vi "自动配置的串口通信组件(Master)vi.vi"(0 "查询":string(combo)="CH0", 5 "error in":errorcluster) -> (14 "读取缓冲区":string, 19 "error out":errorcluster)   [LabVIEW 2013]
uses:
  <vilib>/Instr/_visa.llb/VISA Configure Serial Port (Instr).vi
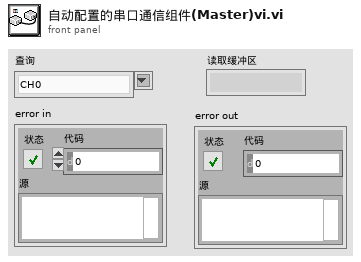
[diagram p1: front panel]
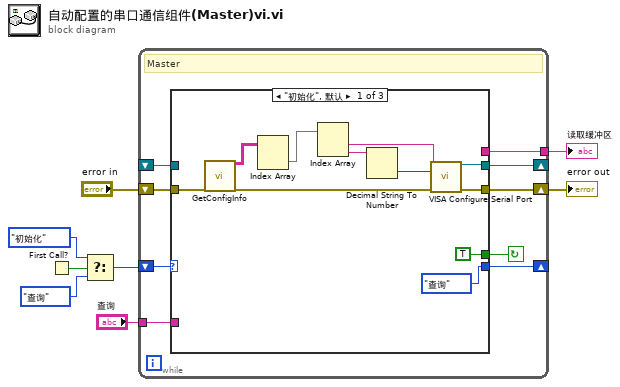
[diagram p0: block diagram]
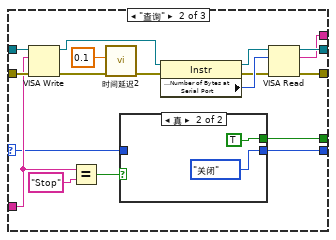
[diagram p2: hidden frame]
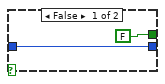
[diagram p3: hidden frame]
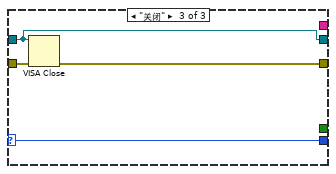
[diagram p4: hidden frame]
diagram:
  n1 = First Call?() -> (First Call?: T/F=w5:bool)
  n2 = Select(t=enum16{"初始化", "空闲", "查询", "关闭"}."初始化" ("枚举"), s=w5, f=enum16{"初始化", "空闲", "查询", "关闭"}."查询" ("枚举")) -> (s? t:f=w4:enum16{"初始化", "空闲", "查询", "关闭"})
  n3 = while {
    shift-right: [w17] -> w1
    shift-left: "error in" -> [w15]
    shift-right: [w16] -> _
    shift-left: _ -> [w14]
    tunnel: "查询" -> [w13]
    tunnel: [w12] -> w7
    shift-right: [w9] -> _
    shift-left: w4 -> [w10]
    stop <- w11 continue-if-true
    # "Master"
    n4 = case shown="\"初始化\", 默认" w10 {
      selector: w10 -> [_ w31 w51]
      tunnel: [w28 w37 w52] -> w16
      tunnel: [w27 w36 w53] -> w17
      tunnel: w15 -> [w24 w38 w54]
      tunnel: w14 -> [_ w39 w52]
      tunnel: w13 -> [_ w34 _]
      tunnel: [_ w35 _] -> w12
      tunnel: [TRUE w29 _] -> w11
      tunnel: [enum16{"初始化", "空闲", "查询", "关闭"}."查询" ("枚举") w30 w51] -> w9
      frame "初始化", Default {
        n5 = call "GetConfigInfo.vi"("error in (no error)"=w24) -> ("串口配置"=w23:string[][], "error out"=w18:errorcluster)  [unwired: 17 in]
        n6 = Index Array(array=w23) -> (element=w22:string[])  [unwired: 2 in]
        n7 = Index Array(array=w22) -> (element #1=w21:string, element #2=w20:string)  [unwired: 2 in]
        n8 = Decimal String To Number(string=w20) -> (number=w19:i32)  [unwired: 2 in, 1 out]
        n9 = call-poly "VISA Configure Serial Port"("VISA resource name"=w21, "baud rate (9600)"=w19, "error in (no error)"=w18) -> ("VISA resource name out"=w28:refnum<visa-resource-name>, "error out"=w27:errorcluster)  [unwired: 11 in]
      }
      frame "查询" {
        n10 = VISA Write(VISA resource name=w39, write buffer=w34, error in (no error)=w38) -> (VISA resource name out=w43:refnum<visa-resource-name>, error out=w41:errorcluster)  [unwired: 1 out]
        n11 = Equal?(x=w34, y="Stop") -> (x = y?=w32:bool)
        n12 = call "时间延迟2"("error in (no error)"=w41, "Delay Time (s)"=0.1) -> ("error out"=w42:errorcluster)  [unwired: 9 in]
        n13 = case shown="真" w32 {
          tunnel: w31 -> [w48 _]
          tunnel: [w48 enum16{"初始化", "空闲", "查询", "关闭"}."关闭"] -> w30
          tunnel: [FALSE TRUE] -> w29
          frame False {
          }
          frame True {
          }
        }
        n14 = property class="Instr"(reference=w43, error in=w42) -> (reference out=w44:refnum<visa-resource-name>, error out=w45:errorcluster, "Serial Settings:Number of Bytes at Serial Port"=w46:u32)
        n15 = VISA Read(VISA resource name=w44, byte count=w46, error in (no error)=w45) -> (VISA resource name out=w37:refnum<visa-resource-name>, read buffer=w35:string, error out=w36:errorcluster)  [unwired: 1 out]
      }
      frame "关闭" {
        n16 = VISA Close(VISA resource name=w52, error in (no error)=w54) -> (error out=w53:errorcluster)
      }
    }
  }
  "读取缓冲区" <- w7
  "error out" <- w1
